vi "Dispatch Start.vi"(8 "error in (no error)":errorcluster) -> (0 "error out":errorcluster, 2 "Execution State Before Start":T1(ring))   [LabVIEW 2014, in "AMC.lvlib"]
uses:
  AMC.lvlib
  _SubVIs/Globals.vi
panel:
  in  "x":u8
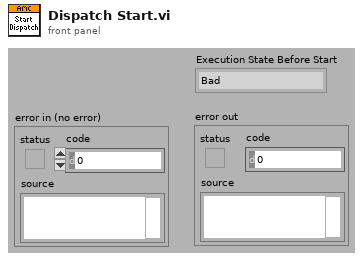
[diagram p1: front panel]
types:
  T1 = enum32{"Bad", "Idle", "Run top level", "Running"}
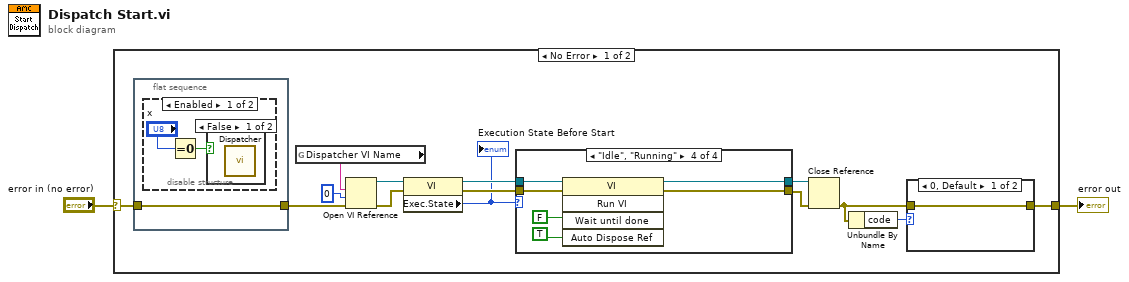
[diagram p0: block diagram]
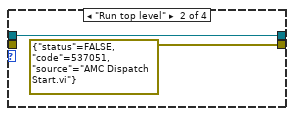
[diagram p3: hidden frame]
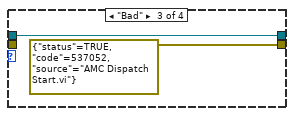
[diagram p4: hidden frame]
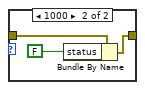
[diagram p7: hidden frame]
diagram:
  n1 = case shown="No Error" "error in (no error)" {
    selector: "error in (no error)" -> [w6 w36]
    tunnel: [w14 w36] -> w2
    frame No Error {
      n2 = flat-sequence {
        tunnel: [w29] -> w9
        tunnel: w6 -> [w29]
        frame #0 {
          n3 = disable-structure shown="Enabled" {
            frame Enabled {
              n4 = Equal To 0?(x="x") -> (x = 0?=w31:bool)
              n5 = case shown="False" w31 {
                frame False {
                  n6 = call "Dispatcher.vi"() -> ()  [unwired: 12 out]
                }
                frame True {
                }
              }
            }
            frame Disabled {
            }
          }
        }
      }
      n7 = global read "Globals.vi" "Dispatcher VI Name"() -> (w3:string)
      n8 = Open VI Reference(vi path=w3, options=0, error in (no error)=w9) -> (vi reference=w11:refnum<vi>, error out=w10:errorcluster)  [unwired: 3 out]
      n9 = property class="VI"(reference=w11, error in=w10) -> (reference out=w8:refnum<vi>, error out=w7:errorcluster, "Exec.State"=w5:T1)
      "Execution State Before Start" <- w5
      n10 = case shown="\"Idle\", \"Running\"" w5 {
        tunnel: [w18 w20 w22 w27] -> w12
        tunnel: [w17 errorcluster {"status"=FALSE, "code"=537051, "source"="AMC Dispatch Start.vi"} ("error out") errorcluster {"status"=TRUE, "code"=537052, "source"="AMC Dispatch Start.vi"} ("error out") w25] -> w4
        tunnel: w8 -> [w18 w20 w22 w24]
        tunnel: w7 -> [w17 _ _ w23]
        frame Default {
        }
        frame "Run top level" {
        }
        frame "Bad" {
        }
        frame "Idle", "Running" {
          n11 = invoke class="VI" method="Run VI"(reference=w24, error in=w23, "Wait until done"=FALSE ("Wait Until Done"), "Auto Dispose Ref"=TRUE) -> (reference out=w27:refnum<vi>, error out=w25:errorcluster)  [unwired: 1 in, 3 out]
        }
      }
      n12 = Close Reference(reference=w12, error in (no error)=w4) -> (error out=w15:errorcluster)
      n13 = Unbundle By Name(w15) -> ("code"=w16:i32)
      n14 = case shown="0, Default" w16 {
        tunnel: w15 -> [w32 w35]
        tunnel: [w32 w34] -> w14
        frame 0, Default {
        }
        frame 1000 {
          n15 = Bundle By Name(cluster=w35, "status"=FALSE) -> (w34:errorcluster)
        }
      }
    }
    frame Error {
    }
  }
  "error out" <- w2
